vi "Configuration File mismatch 6301--error.vi"() -> (0 "error out":errorcluster)   [LabVIEW 2024, in "UI.lvlib"]
uses:
  UI.lvlib
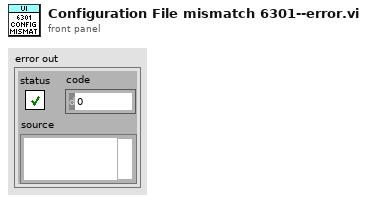
[diagram p1: front panel]
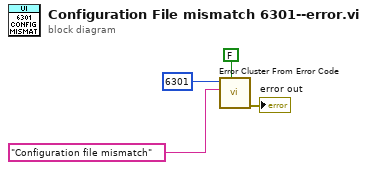
[diagram p0: block diagram]
diagram:
  n1 = call <vilib>:"Error Cluster From Error Code.vi"("show call chain? (False)"=FALSE, "error message (\"\")"="Configuration file mismatch" ("error message (\"\")"), "error code (0)"=6301) -> ("error out"=→"error out":errorcluster)  [unwired: 6 in]
